vi "breakout - kopie.vi"(11 "NXT/EV3":T1) -> (3 "NXT/EV3 2":T1)   [LabVIEW 2013]
uses:
  <vilib>/NXT/Subs/LVHSConnector.ctl
  <vilib>/NXT/LegoClasses/BrickReference/BrickReference.lvclass
  <vilib>/NXT/Dual Mode Library/Display/NXT_Rect.ctl
  <vilib>/NXT/Dual Mode Library/Display/clearDisplay.vi
  <vilib>/NXT/Dual Mode Library/Waits/Wait_Num.vi
  <vilib>/NXT/Dual Mode Library/prims/inRangeAndCoerce/inRangeAndCoerce_float.vi
  <vilib>/NXT/Dual Mode Library/Display/eraseRect.vi
  <vilib>/NXT/Dual Mode Library/Display/drawRect_filled.vi
  <vilib>/NXT/Dual Mode Library/Advanced/NXTFlag_Get_Integer.vi
  <vilib>/NXT/Dual Mode Library/Sensors/EV3_Infrared_Seek.vi
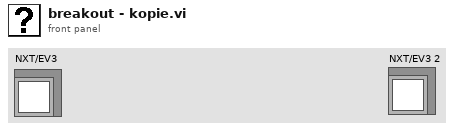
[diagram p1: front panel]
types:
  T1 = typedef "LVHSConnector.ctl" = refnum<class "BrickReference.lvclass">
  T2 = typedef "NXT_Rect.ctl" = cluster{"Left":i16, "Bottom":i16, "Width":i16, "Height":i16}
  T3 = cluster{dbl, dbl, "lower limit":i32, "lower limit":i32}
  T4 = cluster{"Channel 1 Heading":sgl, "Channel 1 Proximity":sgl, "Channel 2 Heading":sgl, "Channel 2 Proximity":sgl, "Channel 3 Heading":sgl, "Channel 3 Proximity":sgl, "Channel 4 Heading":sgl, "Channel 4 Proximity":sgl}
  T5 = cluster{sgl, "Start  Y":i16, "Start  Y":i16, "Start  Y":i16}
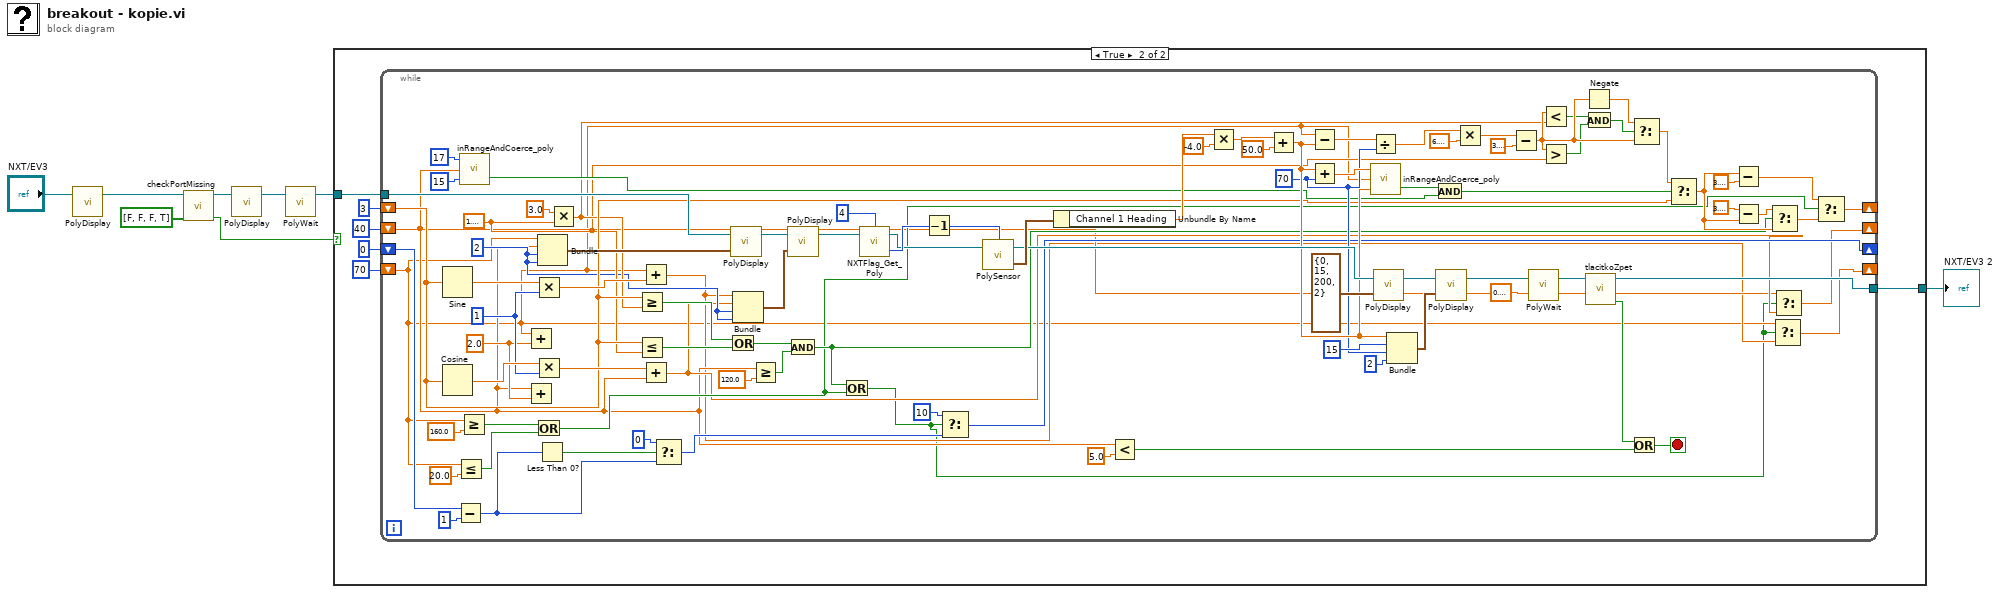
[diagram p0: block diagram]
diagram:
  n1 = call-poly <vilib>:"PolyDisplay.vi"("NXT/EV3"="NXT/EV3") -> ("NXT/EV3"=w7:T1)  [unwired: 3 in]
  n2 = call "checkPortMissing.vi"("Required"=bool[] [FALSE, FALSE, FALSE, TRUE], "NXT/EV3"=w7) -> ("Success"=w5:bool, "NXT/EV3"=w3:T1)  [unwired: 8 in]
  n3 = call-poly <vilib>:"PolyDisplay.vi"("NXT/EV3"=w3) -> ("NXT/EV3"=w1:T1)  [unwired: 3 in]
  n4 = call-poly <vilib>:"PolyWait.vi"("NXT/EV3"=w1) -> ("NXT/EV3"=w2:T1)  [unwired: 3 in]
  n5 = case shown="True" w5 {
    tunnel: [w9 w14] -> w4
    tunnel: w2 -> [w9 w15]
    frame False {
      # "Controllers unavailable"
    }
    frame True {
      n6 = while {
        tunnel: w15 -> [w77]
        tunnel: [w69] -> w14
        shift-right: [w36] -> _
        shift-left: 3 -> [w42]
        shift-right: [w18] -> _
        shift-left: 70 -> [w17]
        shift-right: [w21] -> _
        shift-left: 40 -> [w20]
        shift-right: [w27] -> _
        shift-left: 0 -> [w32]
        stop <- w71 stop-if-true
        w38 = 2 ("lower limit")
        w40 = 1.5707963267948966
        w64 = i16 70 ("Start  Y")
        w82 = 2.0
        w84 = 1
        n7 = Sine(x=w42) -> (sin(x)=w88:dbl)
        n8 = Cosine(x=w42) -> (cos(x)=w87:dbl)
        n9 = Subtract(x=w32, y=1) -> (x-y=w29:i32)
        n10 = Less Or Equal?(x=w17, y=20.0) -> (x <= y?=w49:bool)
        n11 = call-poly <vilib>:"inRangeAndCoerce_poly.vi"("lower limit"=15, "x"=w20, "upper limit"=17) -> ("In Range?"=w61:bool)  [unwired: 1 out]
        n12 = Greater Or Equal?(x=w17, y=160.0) -> (x >= y?=w51:bool)
        n13 = Add(x=w17, y=w82) -> ()  [unwired: 1 out]
        n14 = Add(x=w20, y=w82) -> ()  [unwired: 1 out]
        n15 = Multiply(x=w88, y=w84) -> (x*y=w86:dbl)
        n16 = Multiply(x=w87, y=w84) -> (x*y=w85:dbl)
        n17 = Or(x=w51, y=w49) -> (x .or. y?=w23:bool)
        n18 = Less Than 0?(x=w29) -> (x < 0?=w30:bool)
        n19 = Bundle(w17, w20, "lower limit"=w38, "lower limit"=w38) -> (w78:T3)  [unwired: 1 in]
        n20 = Multiply(x=3.0, y=w40) -> (x*y=w41:dbl)
        n21 = Greater Or Equal?(x=w42, y=w41) -> (x >= y?=w45:bool)
        n22 = Less Or Equal?(x=w42, y=w40) -> (x <= y?=w43:bool)
        n23 = Add(x=w17, y=w86) -> (x+y=w19:dbl)
        n24 = Add(x=w85, y=w20) -> (x+y=w22:dbl)
        n25 = Select(t=0, s=w30, f=w29) -> (s? t:f=w26:i32)
        n26 = Or(x=w45, y=w43) -> (x .or. y?=w44:bool)
        n27 = call-poly <vilib>:"PolyDisplay.vi"("Rect Parameters"=w78, "NXT/EV3"=w77) -> ("NXT/EV3"=w76:T1)  [unwired: 2 in]
        n28 = Bundle(w19, w22, "lower limit"=w38, "lower limit"=w38) -> (w94:T3)  [unwired: 1 in]
        n29 = Greater Or Equal?(x=w20, y=120.0) -> (x >= y?=w48:bool)
        n30 = call-poly <vilib>:"PolyDisplay.vi"("Rect Parameters"=w94, "NXT/EV3"=w76) -> ("NXT/EV3"=w93:T1)  [unwired: 2 in]
        n31 = And(x=w44, y=w48) -> (x .and. y?=w24:bool)
        n32 = Or(x=w24, y=w23) -> (x .or. y?=w16:bool)
        n33 = call-poly <vilib>:"NXTFlag_Get_Poly.vi"("NXT/EV3"=w93, "NXT/EV3 Flag Number"=4) -> ("Flag Value"=w105:i32, "NXT/EV3"=w104:T1)  [unwired: 1 in]
        n34 = Decrement(x=w105) -> (x-1=w103:i32)
        n35 = Select(t=10, s=w16, f=w26) -> (s? t:f=w27:i32)
        n36 = call-poly <vilib>:"PolySensor.vi"("NXT/EV3"=w104, "Port (Port 1)"=w103) -> ("Scaled Values"=w102:T4, "NXT/EV3"=w99:T1)  [unwired: 1 in]
        n37 = Unbundle By Name(w102) -> ("Channel 1 Heading"=w101:sgl)
        n38 = Less?(x=w20, y=5.0) -> (x < y?=w72:bool)
        n39 = Multiply(x=w101, y=sgl -4.0) -> (x*y=w96:sgl)
        n40 = Add(x=w96, y=sgl 50.0) -> (x+y=w65:sgl)
        n41 = Subtract(x=w17, y=w65) -> (x-y=w92:dbl)
        n42 = Add(x=w65, y=w64) -> (x+y=w66:sgl)
        n43 = Divide(x=w92, y=w64) -> (x/y=w90:dbl)
        n44 = call-poly <vilib>:"inRangeAndCoerce_poly.vi"("lower limit"=w65, "x"=w17, "upper limit"=w66) -> ("In Range?"=w63:bool)  [unwired: 1 out]
        n45 = call-poly <vilib>:"PolyDisplay.vi"("Rect Parameters"=T2 {"Left"=0, "Bottom"=15, "Width"=200, "Height"=2}, "NXT/EV3"=w99) -> ("NXT/EV3"=w98:T1)  [unwired: 2 in]
        n46 = Bundle(w65, "Start  Y"=i16 15, "Start  Y"=w64, "Start  Y"=i16 2) -> (w100:T5)  [unwired: 1 in]
        n47 = And(x=w63, y=w61) -> (x .and. y?=w60:bool)
        n48 = call-poly <vilib>:"PolyDisplay.vi"("Rect Parameters"=w100, "NXT/EV3"=w98) -> ("NXT/EV3"=w62:T1)  [unwired: 2 in]
        n49 = Multiply(x=w90, y=6.283185307179586) -> (x*y=w89:dbl)
        n50 = Subtract(x=w89, y=3.141592653589793) -> (x-y=w57:dbl)
        n51 = call-poly <vilib>:"PolyWait.vi"("Time (1 sec)"=sgl 0.1, "NXT/EV3"=w62) -> ("NXT/EV3"=w70:T1)  [unwired: 2 in]
        n52 = Less?(x=w57, y=w41) -> (x < y?=w55:bool)
        n53 = Greater?(x=w57, y=w40) -> (0:w56:bool)
        n54 = Negate(x=w57) -> (-x=w59:dbl)
        n55 = And(x=w55, y=w56) -> (x .and. y?=w54:bool)
        n56 = call "tlacitkoZpet.vi"("NXT/EV3"=w70) -> ("Boolean"=w68:bool, "NXT/EV3 2"=w69:T1)  [unwired: 9 in]
        n57 = Or(x=w68, y=w72) -> (x .or. y?=w71:bool)
        n58 = Select(t=w59, s=w54, f=w57) -> (s? t:f=w58:dbl)
        n59 = Select(t=w58, s=w60, f=w42) -> (s? t:f=w34:dbl)
        n60 = Subtract(x=w34, y=3.141592653589793) -> (x-y=w35:dbl)
        n61 = Subtract(x=3.141592653589793, y=w34) -> (x-y=w39:dbl)
        n62 = Select(t=w39, s=w24, f=w34) -> (s? t:f=w37:dbl)
        n63 = Select(t=w17, s=w16, f=w19) -> (s? t:f=w18:dbl)
        n64 = Select(t=w20, s=w16, f=w22) -> (s? t:f=w21:dbl)
        n65 = Select(t=w35, s=w23, f=w37) -> (s? t:f=w36:dbl)
      }
    }
  }
  "NXT/EV3 2" <- w4
